vi "generate_list_between_bounds.vi"(0 "Upper bound":dbl, 2 "Step size":dbl, 3 "Lower bound":dbl) -> (5 "Array":dbl[](array[numeric]))   [LabVIEW 2019]
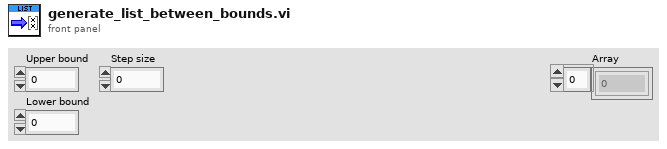
[diagram p1: front panel]
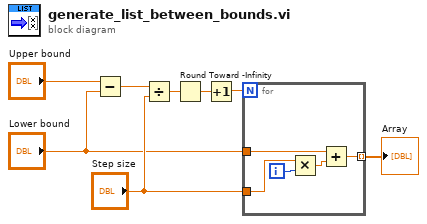
[diagram p0: block diagram]
diagram:
  n1 = Subtract(x="Upper bound", y="Lower bound") -> (x-y=w7:dbl)
  n2 = Divide(x=w7, y="Step size") -> (x/y=w6:dbl)
  n3 = Round Toward -Infinity(1:w6) -> (0:w5:dbl)
  n4 = Increment(x=w5) -> (x+1=w4:dbl)
  n5 = for {
    N: w4 -> [_]
    tunnel: "Step size" -> [w13]
    tunnel: "Lower bound" -> [w10]
    tunnel: [w9] -> w1 mode=indexing
    i -> [w12]
    n6 = Multiply(x=w13, y=w12) -> (x*y=w11:dbl)
    n7 = Add(x=w10, y=w11) -> (x+y=w9:dbl)
  }
  "Array" <- w1
